vi "Calculate Stats from Scrape.vi"() -> (3 "WPC Calculated Player Stats":T1(array[cluster]) {"Calculated Tournament Stats"."Hands Played %" format="%#_3g"; "Calculated Tournament Stats"."Hands Won %" format="%#_3g"; "Calculated Tournament Stats"."Average Hands Dealt Per Tournament" format="%#_4g"; "Calculated Tournament Stats"."Average Hands Won Per Tournament" format="%#_3g"; "Calculated Cash Stats"."Hands Played %" format="%#_3g"; "Calculated Cash Stats"."Hands Won %" format="%#_3g"}, 11 "WPC Player Stats":T2[](array[typedef]) {"Date Updated" format="%<%m/%d/%Y>T"})   [LabVIEW 2020]
uses:
  WPC Player Stats.ctl
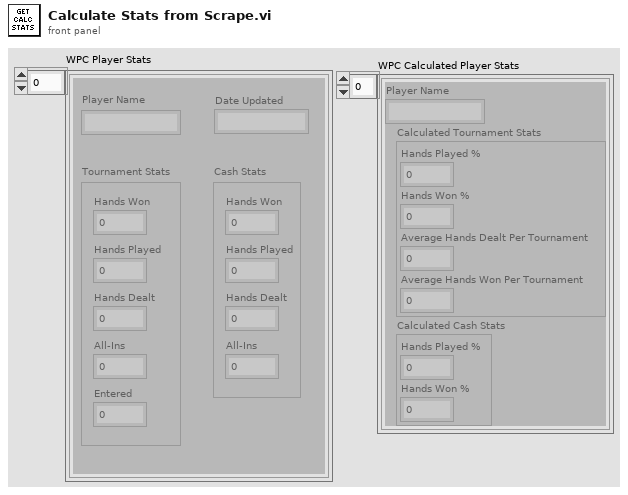
[diagram p1: front panel]
types:
  T1 = cluster{"Player Name":string, "Calculated Tournament Stats":cluster{"Hands Played %":dbl, "Hands Won %":dbl, "Average Hands Dealt Per Tournament":dbl, "Average Hands Won Per Tournament":dbl}, "Calculated Cash Stats":cluster{"Hands Played %":dbl, "Hands Won %":dbl}}[]
  T2 = typedef "WPC Player Stats.ctl" = cluster{"Player Name":string, "Date Updated":timestamp, "Tournament Stats":cluster{"Hands Won":dbl, "Hands Played":dbl, "Hands Dealt":dbl, "All-Ins":dbl, "Entered":dbl}, "Cash Stats":cluster{"Hands Won":dbl, "Hands Played":dbl, "Hands Dealt":dbl, "All-Ins":dbl}}
  T3 = cluster{"Hands Won":dbl, "Hands Played":dbl, "Hands Dealt":dbl, "All-Ins":dbl, "Entered":dbl}
  T4 = cluster{"Hands Won":dbl, "Hands Played":dbl, "Hands Dealt":dbl, "All-Ins":dbl}
  T5 = cluster{"Hands Played %":dbl, "Hands Won %":dbl, "Average Hands Dealt Per Tournament":dbl, "Average Hands Won Per Tournament":dbl}
  T6 = cluster{"Player Name":string, "Calculated Tournament Stats":cluster{"Hands Played %":dbl, "Hands Won %":dbl, "Average Hands Dealt Per Tournament":dbl, "Average Hands Won Per Tournament":dbl}, "Calculated Cash Stats":cluster{"Hands Played %":dbl, "Hands Won %":dbl}}
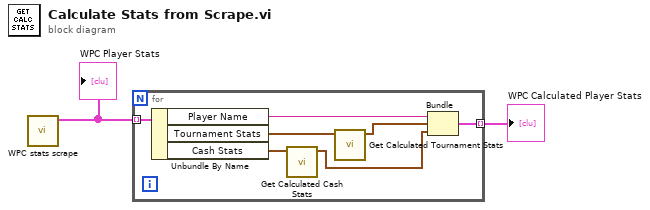
[diagram p0: block diagram]
diagram:
  n1 = call "WPC stats scrape.vi"() -> ("WPC Player Stats"=w2:T2[])  [unwired: 11 in]
  "WPC Player Stats" <- w2
  n2 = for {
    tunnel: w2 -> [w9] mode=indexing
    tunnel: [w3] -> w1 mode=indexing
    n3 = Unbundle By Name(w9) -> ("Player Name"=w6:string, "Tournament Stats"=w8:T3, "Cash Stats"=w7:T4)
    n4 = call "Get Calculated Cash Stats.vi"("Cash Stats"=w7) -> ("Calculated Cash Stats"=w4:cluster{"Hands Played %":dbl, "Hands Won %":dbl})  [unwired: 10 in]
    n5 = call "Get Calculated Tournament Stats.vi"("Tournament Stats"=w8) -> ("Calculated Tournament Stats"=w5:T5)  [unwired: 10 in]
    n6 = Bundle("Player Name"=w6, "Calculated Tournament Stats"=w5, "Calculated Cash Stats"=w4) -> (w3:T6)  [unwired: 1 in]
  }
  "WPC Calculated Player Stats" <- w1
